vi "Multiply by Gain.vi"(8 "error in (no error)":errorcluster, 10 "Gain":dbl[](array[numeric]), 11 "WFM in":waveform(dbl)[](array[waveform])) -> (0 "error out":errorcluster, 3 "WFM out":waveform(dbl)[](array[waveform]))   [LabVIEW 2019, in "Instrument.Lockin.lvclass"]
uses:
  Instrument.Lockin.lvclass
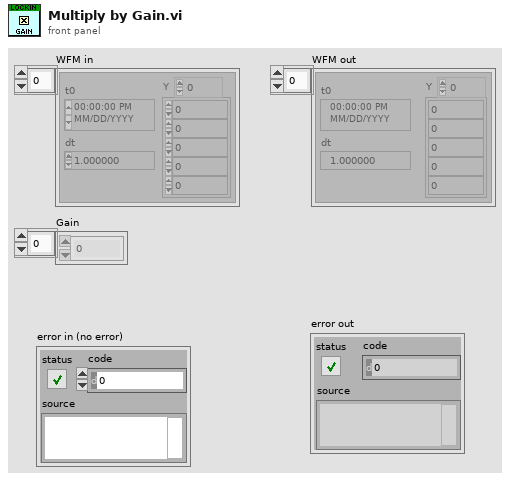
[diagram p1: front panel]
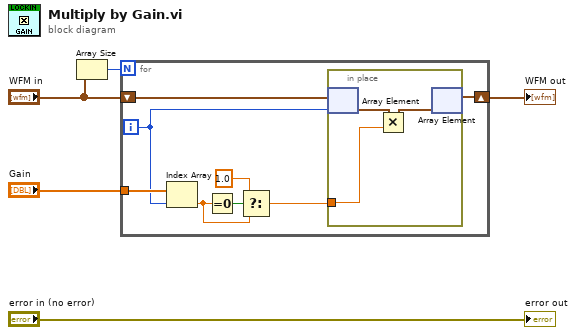
[diagram p0: block diagram]
diagram:
  n1 = Array Size(array="WFM in") -> (size(s)=w5:i32)
  n2 = for {
    N: w5 -> [_]
    shift-right: [w12] -> w4
    shift-left: "WFM in" -> [w13]
    tunnel: "Gain" -> [w11]
    i -> [w10]
    n3 = Index Array(array=w11, index=w10) -> (element=w7:dbl)
    n4 = Equal To 0?(x=w7) -> (x = 0?=w9:bool)
    n5 = Select(t=1.0, s=w9, f=w7) -> (s? t:f=w6:dbl)
    n6 = in-place {
      in-place-border: w6 -> [w15]
      n7 = in-place-array #1(w13, w10) -> (w16:waveform(dbl))
      n8 = Multiply(x=w16, y=w15) -> (x*y=w14:waveform(dbl))
      n9 = in-place-array #1(w14) -> (w12:waveform(dbl)[])  [unwired: 1 out]
    }
  }
  "WFM out" <- w4
  "error out" <- "error in (no error)"
